vi "1_2_Duality principle.vi"() -> ()   [LabVIEW 2009]
uses:
  <vilib>/Analysis/2dsp.llb/Inverse Complex FFT.vi
  <vilib>/Analysis/2dsp.llb/Complex FFT.vi
  <vilib>/Analysis/2dsp.llb/Real FFT.vi
  <vilib>/Analysis/NI_AALBase.lvlib
  <vilib>/Analysis/NI_AALPro.lvlib
panel:
  in  "stop":bool
  out "Frequency domain":dbl[](graph)=[0.01, 0.0, 0.0, 0.0, 0.0, 0.0, 0.0, 0.0, 0.0, 0.0, 0.0, 0.0, 0.0, 0.0, 0.0, 0.0, 0.0, 0.0, 0.0, 0.0, 0.0, 0.0, 0.0, 0.0, 0.0, 0.0, 0.0, 0.0, 0.0, 0.0, 0.0, 0.0, 0.0, 0.0, 0.0, 0.0, 0.0, 0.0, 0.0, 0.0, 0.0, 0.0, 0.0, 0.0, 0.0, 0.0, 0.0, 0.0, 0.0, 0.0, 0.0, 0.0, 0.0, 0.0, 0.0, 0.0, 0.0, 0.0, 0.0, 0.0, 0.0, 0.0, 0.0, 0.0, 0.0, 0.0, 0.0, 0.0, 0.0, 0.0, 0.0, 0.0, 0.0, 0.0, 0.0, 0.0, 0.0, 0.0, 0.0, 0.0, 0.0, 0.0, 0.0, 0.0, 0.0, 0.0, 0.0, 0.0, 0.0, 0.0, 0.0, 0.0, 0.0, 0.0, 0.0, 0.0, 0.0, 0.0, 0.0, 0.0]
  out "Time domain":dbl[](graph)=[0.01, 0.01, 0.01, 0.01, 0.01, 0.01, 0.01, 0.01, 0.01, 0.01, 0.01, 0.01, 0.01, 0.01, 0.01, 0.01, 0.01, 0.01, 0.01, 0.01, 0.01, 0.01, 0.01, 0.01, 0.01, 0.01, 0.01, 0.01, 0.01, 0.01, 0.01, 0.01, 0.01, 0.01, 0.01, 0.01, 0.01, 0.01, 0.01, 0.01, 0.01, 0.01, 0.01, 0.01, 0.01, 0.01, 0.01, 0.01, 0.01, 0.01, 0.01, 0.01, 0.01, 0.01, 0.01, 0.01, 0.01, 0.01, 0.01, 0.01, 0.01, 0.01, 0.01, 0.01, 0.01, 0.01, 0.01, 0.01, 0.01, 0.01, 0.01, 0.01, 0.01, 0.01, 0.01, 0.01, 0.01, 0.01, 0.01, 0.01, 0.01, 0.01, 0.01, 0.01, 0.01, 0.01, 0.01, 0.01, 0.01, 0.01, 0.01, 0.01, 0.01, 0.01, 0.01, 0.01, 0.01, 0.01, 0.01, 0.01]
  out "Frequency domain":dbl[](graph)=[0.0, 0.0, 0.0, 0.0, 0.0, 0.0, 0.0, 0.0, 0.0, 0.0, 1.0, 0.0, 0.0, 0.0, 0.0, 0.0, 0.0, 0.0, 0.0, 0.0, 0.0, 0.0, 0.0, 0.0, 0.0, 0.0, 0.0, 0.0, 0.0, 0.0, 0.0, 0.0, 0.0, 0.0, 0.0, 0.0, 0.0, 0.0, 0.0, 0.0, 0.0, 0.0, 0.0, 0.0, 0.0, 0.0, 0.0, 0.0, 0.0, 0.0, 0.0, 0.0, 0.0, 0.0, 0.0, 0.0, 0.0, 0.0, 0.0, 0.0, 0.0, 0.0, 0.0, 0.0, 0.0, 0.0, 0.0, 0.0, 0.0, 0.0, 0.0, 0.0, 0.0, 0.0, 0.0, 0.0, 0.0, 0.0, 0.0, 0.0, 0.0, 0.0, 0.0, 0.0, 0.0, 0.0, 0.0, 0.0, 0.0, 0.0, 0.0, 0.0, 0.0, 0.0, 0.0, 0.0, 0.0, 0.0, 0.0, 0.0]
  out "Time domain":dbl[](graph)=[0.0198, 0.0002, 0.0002, 0.0002, 0.0002, 0.0002, 0.0002, 0.0002, 0.0002, 0.0002, 0.00019999999999999727, 0.0002, 0.0002, 0.0002, 0.0002, 0.0002, 0.0002, 0.0002, 0.0002, 0.0002, 0.00019999999999999977, 0.0002, 0.0002, 0.0002, 0.0002, 0.0002, 0.0002, 0.0002, 0.0002, 0.0002, 0.00019999999999999977, 0.0002, 0.0002, 0.0002, 0.0002, 0.0002, 0.0002, 0.0002, 0.0002, 0.0002, 0.00019999999999999727, 0.0002, 0.0002, 0.0002, 0.0002, 0.0002, 0.0002, 0.0002, 0.0002, 0.0002]
  out "Frequency domain":dbl[](graph)=[0.01, 0.02, 0.019999999999999997, 0.019999999999999997, 0.02, 0.02, 0.02, 0.019999999999999997, 0.019999999999999997, 0.02, 0.02, 0.02, 0.019999999999999997, 0.019999999999999997, 0.02, 0.02, 0.02, 0.019999999999999997, 0.019999999999999997, 0.02, 0.02, 0.02, 0.019999999999999997, 0.019999999999999997, 0.02, 0.02, 0.02, 0.019999999999999997, 0.019999999999999997, 0.02, 0.02, 0.02, 0.019999999999999997, 0.019999999999999997, 0.02, 0.02, 0.02, 0.019999999999999997, 0.019999999999999997, 0.02, 0.02, 0.02, 0.019999999999999997, 0.019999999999999997, 0.02, 0.02, 0.02, 0.019999999999999997, 0.019999999999999997, 0.02]
  in  "Samples":dbl=100.0
  out "Time domain":dbl[](graph)=[0.0, 0.0, 0.0, 0.0, 0.0, 0.0, 0.0, 0.0, 0.0, 0.0, 1.0, 0.0, 0.0, 0.0, 0.0, 0.0, 0.0, 0.0, 0.0, 0.0, 0.0, 0.0, 0.0, 0.0, 0.0, 0.0, 0.0, 0.0, 0.0, 0.0, 0.0, 0.0, 0.0, 0.0, 0.0, 0.0, 0.0, 0.0, 0.0, 0.0, 0.0, 0.0, 0.0, 0.0, 0.0, 0.0, 0.0, 0.0, 0.0, 0.0, 0.0, 0.0, 0.0, 0.0, 0.0, 0.0, 0.0, 0.0, 0.0, 0.0, 0.0, 0.0, 0.0, 0.0, 0.0, 0.0, 0.0, 0.0, 0.0, 0.0, 0.0, 0.0, 0.0, 0.0, 0.0, 0.0, 0.0, 0.0, 0.0, 0.0, 0.0, 0.0, 0.0, 0.0, 0.0, 0.0, 0.0, 0.0, 0.0, 0.0, 0.0, 0.0, 0.0, 0.0, 0.0, 0.0, 0.0, 0.0, 0.0, 0.0]
  in  "Delay":dbl(slide)=10.0 scale=0.0..100.0
  # "PRINCIPLE OF DUALITY"
  # "INVERSE FOURIER TRANSFORM"
  # "FOURIER TRANSFORM"
  # "TIME DOMAIN TO FREQUENCY DOMAIN AND BACK TO TIME DOMAIN"
  # "FREQUENCY DOMAIN TO TIME DOMAIN AND BACK TO FREQUENCY DOMAIN"
  # "INVERSE FOURIER TRANSFORM"
  # "FOURIER TRANSFORM"
  # "Program developed by Indranil Sinharoy"
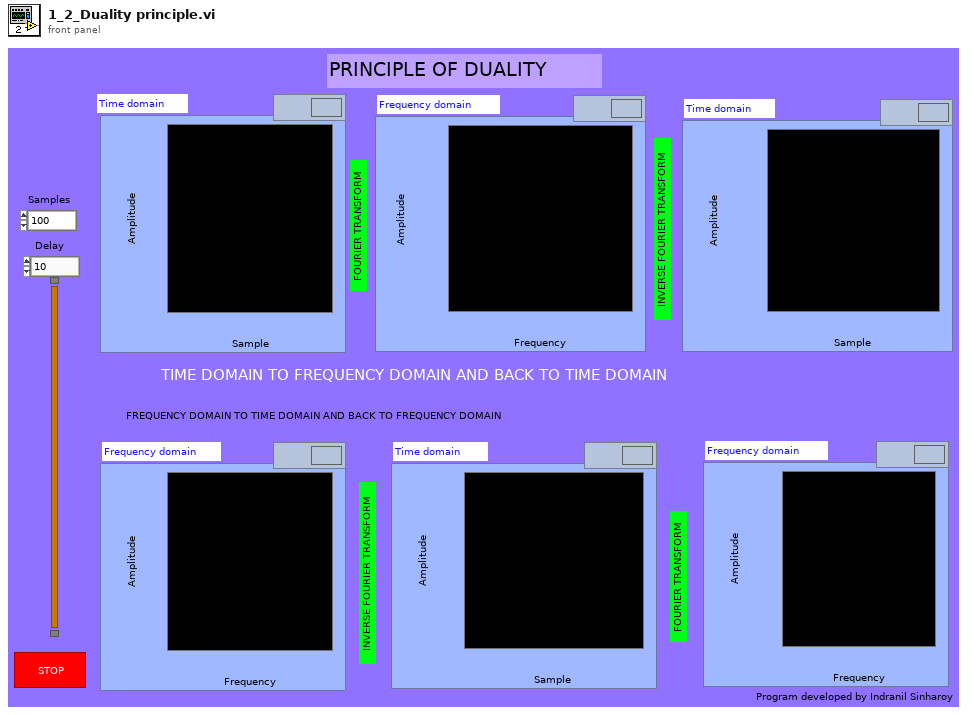
[diagram p1: front panel]
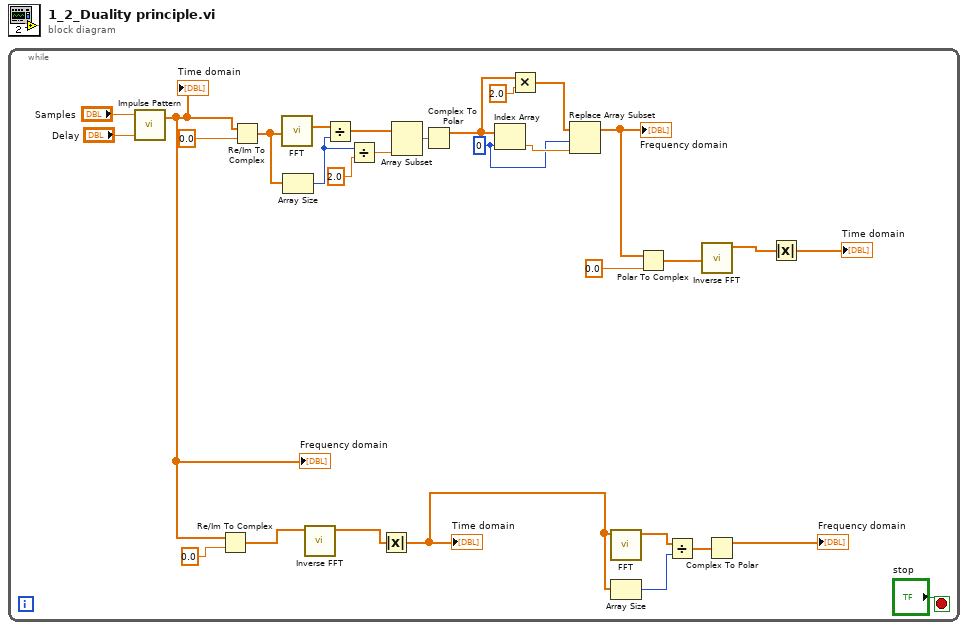
[diagram p0: block diagram]
diagram:
  n1 = while {
    stop <- "stop" stop-if-true
    w19 = 0 ("index")
    n2 = call <vilib>:"Impulse Pattern.vi"("delay"="Delay", "samples"="Samples") -> ("Impulse Pattern"=w9:dbl[])  [unwired: 1 in, 1 out]
    "Time domain" <- w9
    "Frequency domain" <- w9
    n3 = Re/Im To Complex(1:0.0, 2:w9) -> (0:w8:cdb[])
    n4 = Re/Im To Complex(1:0.0, 2:w9) -> (0:w26:cdb[])
    n5 = call-poly <vilib>:"FFT.vi"("X"=w26) -> ("FFT {X}"=w27:cdb[])  [unwired: 9 in, 1 out]
    n6 = Array Size(array=w26) -> (size(s)=w23:i32)
    n7 = call-poly <vilib>:"Inverse FFT.vi"("FFT {X}"=w8) -> ("X"=w10:cdb[])  [unwired: 9 in, 1 out]
    n8 = Divide(x=w27, y=w23) -> (x/y=w25:cdb[])
    n9 = Divide(x=w23, y=2.0) -> (x/y=w24:dbl)
    n10 = Absolute Value(x=w10) -> (abs(x)=w5:dbl[])
    "Time domain" <- w5
    n11 = Array Subset(array=w25, length=w24) -> (w21:cdb[])  [unwired: 1 in]
    n12 = Complex To Polar(r * e^(i*theta)=w21) -> (r=w11:dbl[])  [unwired: 1 out]
    n13 = Index Array(array=w11, index=w19) -> (element=w20:dbl)
    n14 = Multiply(x=w11, y=2.0) -> (x*y=w17:dbl[])
    n15 = Replace Array Subset(array=w17, new element=w20, index=w19) -> (w16:dbl[])
    "Frequency domain" <- w16
    n16 = call-poly <vilib>:"FFT.vi"("X"=w5) -> ("FFT {X}"=w6:cdb[])  [unwired: 9 in, 1 out]
    n17 = Array Size(array=w5) -> (size(s)=w4:i32)
    n18 = Polar To Complex(1:0.0, 2:w16) -> (0:w14:cdb[])
    n19 = Divide(x=w6, y=w4) -> (x/y=w3:cdb[])
    n20 = call-poly <vilib>:"Inverse FFT.vi"("FFT {X}"=w14) -> ("X"=w13:cdb[])  [unwired: 9 in, 1 out]
    n21 = Complex To Polar(r * e^(i*theta)=w3) -> (r=→"Frequency domain":dbl[])  [unwired: 1 out]
    n22 = Absolute Value(x=w13) -> (abs(x)=→"Time domain":dbl[])
  }
